vi "LEIN CMD send ACTI f2 reset error.vi"(0 "Master":u8=42, 1 "Retry on err (F)":bool, 2 "Via master":bool, 5 "SID":u8=42, 7 "LEIN Variation":T1=enum."LEIN63", 11 "error in (no error)":errorcluster) -> (15 "error out":errorcluster)   [LabVIEW 2011]
uses:
  Defenitions/LEIN Structure variations.ctl
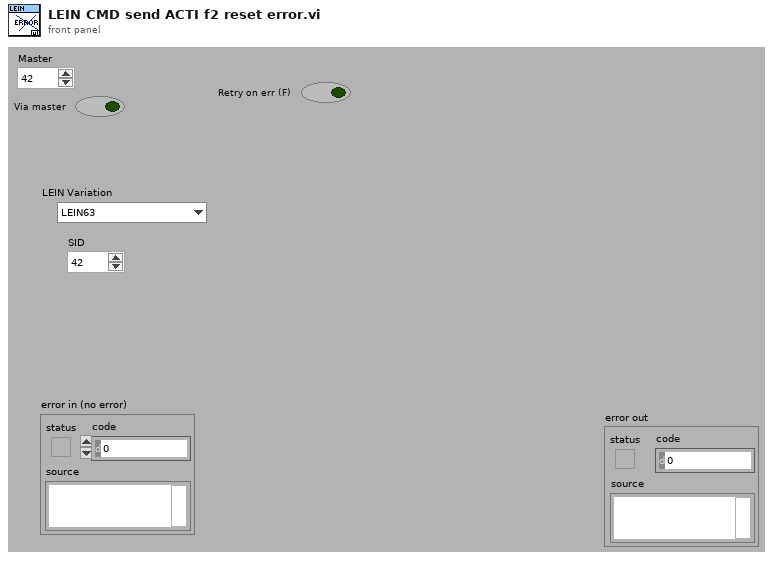
[diagram p1: front panel]
types:
  T1 = typedef "LEIN Structure variations.ctl" = enum16{"LEIN08", "LEIN31", "LEIN63"}
  T2 = typedef "LEIN CMD Cluster.ctl" = cluster{"SID":u8, "ANF":bool, "CMD":T3, "DATA":u8[]}
  T3 = typedef "LEIN CMD List.ctl" = enum8{"ACTI", "TASK", "RES0", "STAT", "RES1", "RES2", "RES3", "USER"}
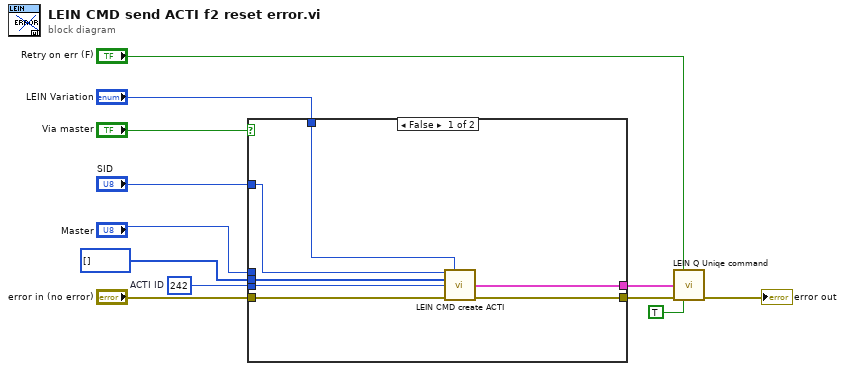
[diagram p0: block diagram]
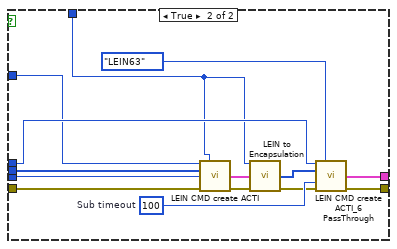
[diagram p2: hidden frame]
diagram:
  w4 = u8 242  # ACTI ID
  n1 = case shown="False" "Via master" {
    tunnel: "LEIN Variation" -> [w19 w20]
    tunnel: [w18 w25] -> w10
    tunnel: [w17 w26] -> w9
    tunnel: "Master" -> [_ w24]
    tunnel: "error in (no error)" -> [w16 w27]
    tunnel: w4 -> [w15 w22]
    tunnel: u8[] [] ("Data") -> [w14 w21]
    tunnel: "SID" -> [w13 w23]
    frame False {
      n2 = call "LEIN CMD create ACTI.vi"("SID"=w13, "LEIN Variation"=w19, "Data"=w14, "ACTI ID"=w15, "error in (no error)"=w16) -> ("CMD"=w18:T2, "error out"=w17:errorcluster)  [unwired: 9 in]
    }
    frame True {
      w31 = u16 100  # Sub timeout
      n3 = call "LEIN CMD create ACTI.vi"("SID"=w23, "LEIN Variation"=w20, "Data"=w21, "ACTI ID"=w22, "error in (no error)"=w27) -> ("CMD"=w33:T2, "error out"=w32:errorcluster)  [unwired: 9 in]
      n4 = call "LEIN to Encapsulation.vi"("LEIN Variation"=w20, "CMD"=w33, "error in (no error)"=w32) -> ("Data and header"=w30:u8[], "error out"=w29:errorcluster)  [unwired: 8 in, 3 out]
      n5 = call "LEIN CMD create ACTI_6 PassThrough.vi"("SID"=w24, "LEIN Variation"=LEIN_Structure_variations."LEIN63", "LEIN ecapsulated data (header and data)"=w30, "Sub Timeout (ms)"=w31, "error in (no error)"=w29) -> ("CMD"=w25:T2, "error out"=w26:errorcluster)  [unwired: 9 in]
    }
  }
  n6 = call "LEIN Q Uniqe command.vi"("Retry on err (F)"="Retry on err (F)", "CMD"=w10, "error in"=w9, "priority(F)"=TRUE) -> ("error out"=→"error out":errorcluster)  [unwired: 11 in]
